vi "SpareRelay(DPDT)_separated.vi"(10 "Array(4)":bool[](array[boolean]), 11 "Mem_mapping in":u16[](array[numeric])) -> (3 "Mem Mapping out":u16[](array[numeric]))   [LabVIEW 2018, in "MB Relay.lvlib"]
uses:
  MB Relay.lvlib
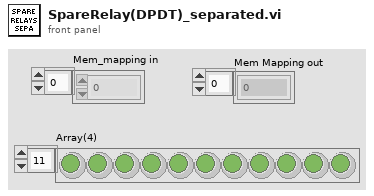
[diagram p1: front panel]
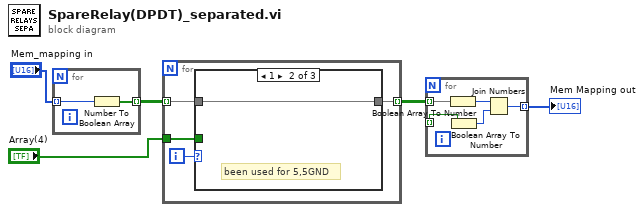
[diagram p0: block diagram]
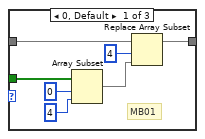
[diagram p2: hidden frame]
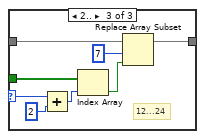
[diagram p3: hidden frame]
diagram:
  n1 = for {
    tunnel: [w7] -> w4 mode=indexing
    tunnel: "Mem_mapping in" -> [w6] mode=indexing
    n2 = Number To Boolean Array(number=w6) -> (Boolean array=w7:bool[])
  }
  n3 = for {
    tunnel: w4 -> [w10] mode=indexing
    tunnel: "Array(4)" -> [w9]
    tunnel: [w8] -> w3 mode=indexing
    i -> [w11]
    n4 = case shown="1" w11 {
      selector: w11 -> [_ _ w26]
      tunnel: w10 -> [w15 w19 w23]
      tunnel: w9 -> [w18 _ w27]
      tunnel: [w12 w19 w20] -> w8
      frame 0, Default {
        # "MB01"
        n5 = Array Subset(array=w18, index=0, length=4) -> (w14:bool[])
        n6 = Replace Array Subset(array=w15, new element=w14, index=4) -> (w12:bool[])
      }
      frame 1 {
        # "been used for 5,5GND"
      }
      frame 2.. {
        # "12...24"
        n7 = Add(x=w26, y=2) -> (x+y=w24:i32)
        n8 = Index Array(array=w27, index=w24) -> (element=w21:bool)
        n9 = Replace Array Subset(array=w23, new element=w21, index=7) -> (w20:bool[])
      }
    }
  }
  n10 = for {
    tunnel: w3 -> [w32] mode=indexing
    tunnel: _ -> [w31] mode=indexing
    tunnel: [w28] -> w2 mode=indexing
    n11 = Boolean Array To Number(Boolean array=w32) -> (number=w30:u8)
    n12 = Boolean Array To Number(Boolean array=w31) -> (number=w29:u8)
    n13 = Join Numbers(hi=w30, lo=w29) -> ((hi.lo)=w28:u16)
  }
  "Mem Mapping out" <- w2
